vi "Main_lv_documentation.vi"(8 "error in (no error)":errorcluster, 11 "VI path":path) -> (0 "error out":errorcluster)   [LabVIEW 2020, in "lv_documentation.lvlib"]
uses:
  lv_documentation.lvlib
  src/models/llm_gemini_chatmodels/llm_gemini_chatmodels.lvclass
  D:/labview-llm-libraries/labview-llm-libraries/src/models/abstract_llm_base/abstract_llm_base.lvclass
  src/models/message_image/message_image.lvclass
  D:/labview-llm-libraries/labview-llm-libraries/src/models/abstract_message_base/abstract_message_base.lvclass
  src/models/message_image/create_image_message.vi
  src/models/llm_gemini_chatmodels/Instantiate_llm_gemini.vi
  src/models/message_text/get_text_message_value.vi
  src/models/abstract_llm_chatcompletion/abstract_llm_chatcompletion.lvclass
  src/models/message_text/message_text.lvclass
panel:
  out "Documentation":string
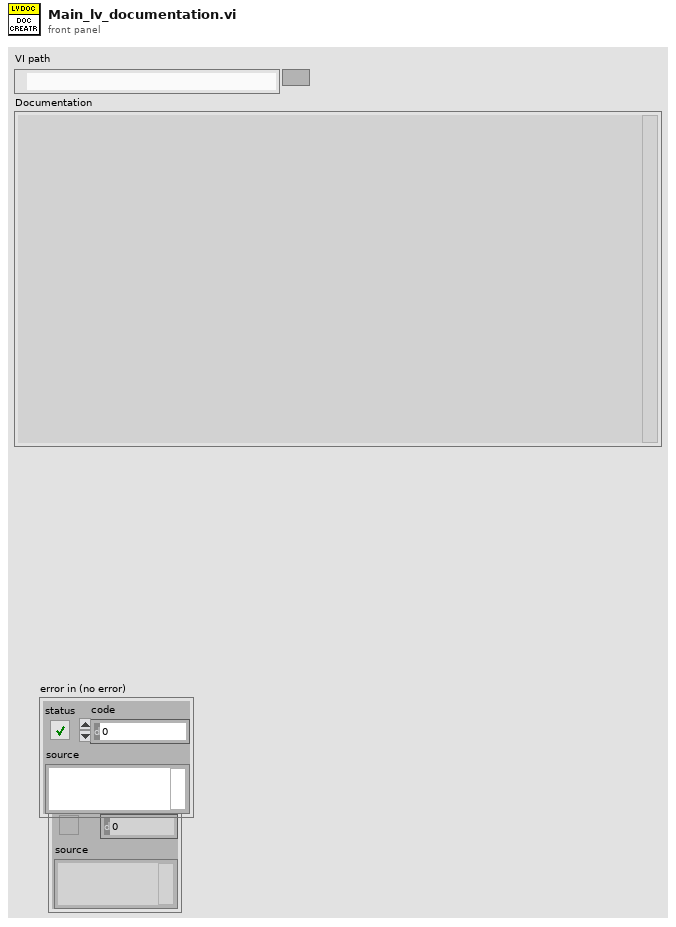
[diagram p1: front panel]
types:
  T1 = cluster{"Documentation":string, "ControlDetails":cluster{"ControlName":string, "Description":string, "TipStrip":string}[], "VIDescription":string}
  T2 = cluster{"ControlName":string, "Description":string, "TipStrip":string}[]
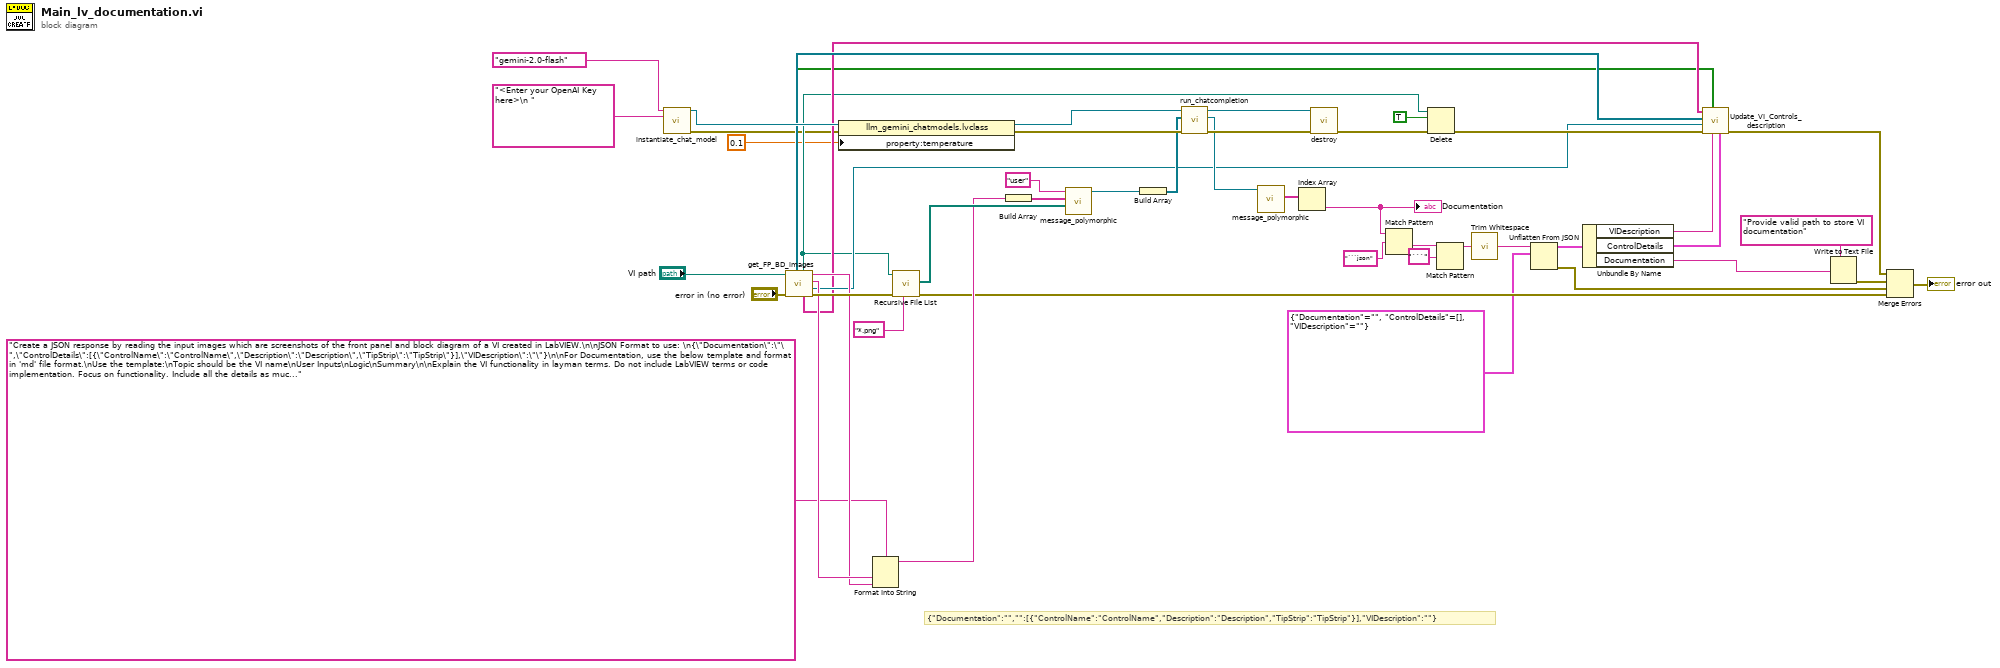
[diagram p0: block diagram]
diagram:
  # "{\"Documentation\":\"\",\"\":[{\"ControlName\":\"ControlName\",\"Description\":\"Description\",\"TipStrip\":\"TipStrip\"}],\"VIDescription\":\"\"}"
  n1 = call-poly "instantiate_chat_model.vi"("model_name"="gemini-2.0-flash", "Gemini_api_key"="<Enter your OpenAI Key here>\n ") -> ("llm_openai out"=w48:refnum<class "llm_gemini_chatmodels.lvclass">, "error out"=w4:errorcluster)  [unwired: 12 in]
  n2 = call "get_FP_BD_images.vi"("error in (no error)"="error in (no error)", "VI Path"="VI path") -> ("error out"=w36:errorcluster, "VI Ref"=w30:refnum<vi>, "VI Name"=w33:string, "Control details"=w32:string, "Control Labels"=w28:string[], "Images Folder"=w27:path, "Control References"=w29:refnum<vi>[], "Indicator/Control"=w1:bool[])  [unwired: 2 in]
  n3 = property class="llm_gemini_chatmodels.lvclass"(reference=w48, error in=w4, "property:temperature"=0.1) -> (reference out=w46:refnum<class "llm_gemini_chatmodels.lvclass">, error out=w47:errorcluster)
  n4 = Format Into String(format string="Create a JSON response by reading the input images which are screenshots of the front panel and block diagram of a VI created in LabVIEW.\n\nJSON Format to use: \n{\"Documentation\":\"\",\"ControlDetails\":[{\"ControlName\":\"ControlName\",\"Description\":\"Description\",\"TipStrip\":\"TipStrip\"}],\"VIDescription\":\"\"}\n\nFor Documentation, use the below template and format in 'md' file format.\nUse the template:\nTopic should be the VI name\nUser Inputs\nLogic\nSummary\n\nExplain the VI functionality in layman terms. Do not include LabVIEW terms or code implementation. Focus on functionality. Include all the details as much as possible.\nDo not include any intro sentence or response to the request.\n\nVI Name is '%s'.\n\nFor Control name, description and tip strip, below are the existing details. Modify if irrelevant or not proper.\n%s\n\nThe tip strips should not exceed 200 characters. Description should not exceed 500 characters. Form this under separate section titled 'ControlDocumentation'. Description should be specific to developer. Tip Strip should be for the user.\n\nMake VIDescription not more than 1000 characters.\n\n" ("text"), w33, w32) -> (resulting string=w31:string)  [unwired: 2 in, 1 out]
  n5 = call <vilib>:"Recursive File List.vi"("pattern"="*.png", "error in (no error)"=w36, "Folder Path"=w27) -> ("error out"=w24:errorcluster, "All Files in Dir"=w40:path[])  [unwired: 4 in, 3 out]
  n6 = Build Array(w31) -> (w39:string[])
  n7 = call-poly "message_polymorphic.vi"("images"=w40, "text"=w39, "role"="user") -> ("message_text out"=w42:refnum<class "message_image.lvclass">)  [unwired: 7 in, 1 out]
  n8 = Build Array(w42) -> (w38:refnum<class "message_image.lvclass">[])
  n9 = call "run_chatcompletion.vi"("error in (no error)"=w47, "Messages"=w38, "abstract_llm_chatcompletion in"=w46) -> ("error out"=w44:errorcluster, "Response"=w43:refnum<class "abstract_message_base.lvclass">, "abstract_llm_chatcompletion out"=w45:refnum<class "llm_gemini_chatmodels.lvclass">)  [unwired: 6 in]
  n10 = call-poly "message_polymorphic.vi"("abstract_message_base.lvclass"=w43) -> ("content"=w49:string[])  [unwired: 8 in, 2 out]
  n11 = Index Array(array=w49) -> (element=w3:string)  [unwired: 1 in]
  "Documentation" <- w3
  n12 = call-dynamic "destroy.vi"("error in (no error)"=w44, "abstract_llm_base in"=w45) -> ("error out"=w35:errorcluster)  [unwired: 8 in, 1 out]
  n13 = Match Pattern(string=w3, regular expression="```json") -> (after substring=w19:string)  [unwired: 1 in, 3 out]
  n14 = Delete(path (use dialog)=w27, entire hierarchy (F)=TRUE, error in=w35) -> (error out=w34:errorcluster)  [unwired: 2 in, 2 out]
  n15 = Match Pattern(string=w19, regular expression="```") -> (before substring=w17:string)  [unwired: 1 in, 3 out]
  n16 = call <vilib>:"Trim Whitespace.vi"("string"=w17) -> ("trimmed string"=w11:string)  [unwired: 1 in]
  n17 = Unflatten From JSON(JSON string=w11, type and defaults=T1 {"Documentation"="", "ControlDetails"=[], "VIDescription"=""}) -> (value=w15:T1, error out=w12:errorcluster)  [unwired: 5 in]
  n18 = Unbundle By Name(w15) -> ("VIDescription"=w2:string, "ControlDetails"=w13:T2, "Documentation"=w14:string)
  n19 = call "Update_VI_Controls_description.vi"("ControlDetails"=w13, "VI Description"=w2, "Indicator/Control"=w1, "error in (no error)"=w34, "VI Ref"=w30, "Control References"=w29, "Control Labels"=w28) -> ("error out"=w23:errorcluster)  [unwired: 4 in]
  n20 = Write to Text File(prompt (Choose or enter file path)="Provide valid path to store VI documentation", text=w14) -> (error out=w25:errorcluster)  [unwired: 2 in, 2 out]
  n21 = Merge Errors(w23, w25, w12, w24) -> (→"error out":errorcluster)
